vi "NI_FPGA_PPG.get FPGA clock.vi"(0 "i ref in":refnum<vi>, 5 "error in (no error)":errorcluster) -> (14 "i ref out":refnum<vi>, 16 "clockRate [ticks/us]":dbl, 19 "error out":errorcluster)   [LabVIEW 2014, in "NI_FPGA_PPG.lvlib"]
doc: "Gets the clock rate of the FPGA."
uses:
  NI_FPGA_PPG.lvlib
  instr.lib/NI-FPGA-PPG/host/instrumentDriver/NI-FPGA-PPG_Driver.lvlib
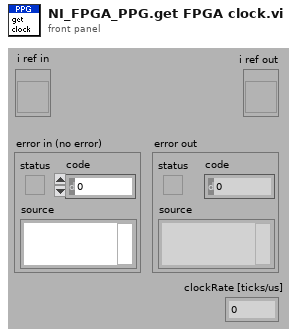
[diagram p1: front panel]
types:
  T1 = typedef "NI_FPGA_PPG.lvlib/NI_FPGA_PPG.i attribute.ctl" = cluster{"dim_service_id":cluster{"dim_actual_device_status":i32, "dim_event_data":i32, "dim_cmd_data":i32, "dim_cmd_data _description":i32, "dim_channel_description":i32}, "VISA":refnum<visa-resource-name>, "actual_device_status":i32, "event_data_id":i32, "pdc_enabled":bool, "pdc_timestamp":u32, "cmd_data_string":string, "cmd_data_size":i32, "cmd_data_description_string":string, "cmd_data_description_size":i32, "channel_description_string":string, "channel_description_size":i32}
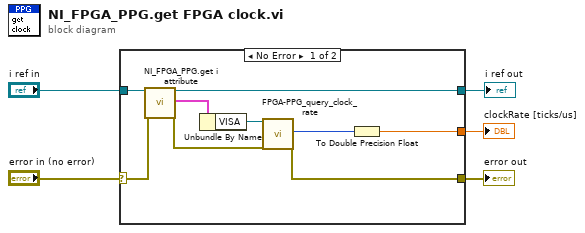
[diagram p0: block diagram]
diagram:
  n1 = case shown="No Error" "error in (no error)" {
    selector: "error in (no error)" -> [w13 w15]
    tunnel: "i ref in" -> [w14 w16]
    tunnel: [w9 w16] -> w3
    tunnel: [w7 _] -> w2
    tunnel: [w6 w15] -> w1
    frame No Error {
      n2 = call "NI_FPGA_PPG.get i attribute.vi"("i ref in"=w14, "error in (no error)"=w13) -> ("i ref out"=w9:refnum<vi>, "i attribute"=w12:T1, "error out"=w10:errorcluster)  [unwired: 15 in]
      n3 = Unbundle By Name(w12) -> ("VISA"=w11:refnum<visa-resource-name>)
      n4 = call "FPGA-PPG_query_clock_rate.vi"("resource_in"=w11, "error in (no error)"=w10) -> ("clockRate [ticks/us]"=w8:i32, "error out"=w6:errorcluster)  [unwired: 15 in, 1 out]
      n5 = To Double Precision Float(number=w8) -> (double precision float=w7:dbl)
    }
    frame Error {
    }
  }
  "error out" <- w1
  "clockRate [ticks/us]" <- w2
  "i ref out" <- w3
